vi "Set flow control 0_none.vi"(8 "error in (no error)":errorcluster caption="entrée d'erreur (pas d'erreur)", 10 "flow control (0:none)":u16(ring) items=["Aucun", "XON/XOFF", "RTS/CTS", "XON/XOFF & RTS/CTS", "DTR/DSR", "XON/XOFF & DTR/DSR"], 11 "Class Instrument UART en entrée":refnum<class "Class Instrument UART.lvclass">) -> (0 "error out":errorcluster caption="sortie d'erreur", 3 "Class Instrument UART en sortie":refnum<class "Class Instrument UART.lvclass">)   [LabVIEW 2020, in "Library Instrument & Equipement.lvlib" / "Library Instruments.lvlib" / "Class Instrument UART.lvclass"]
uses:
  Class Instrument UART.lvclass
  Class Instrument UART.lvclass/Class Instrument UART.ctl
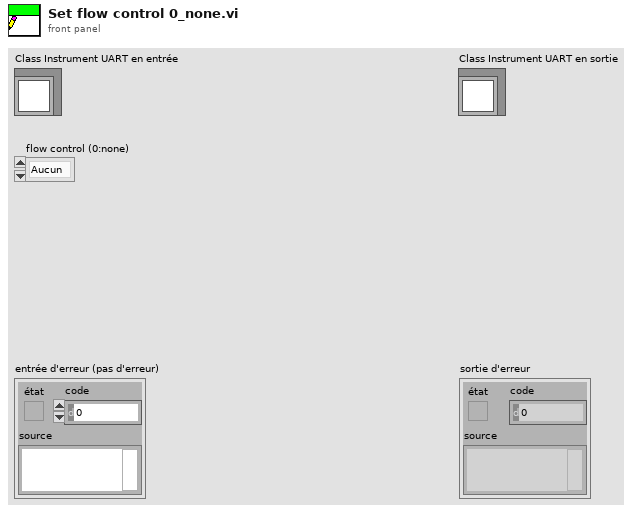
[diagram p1: front panel]
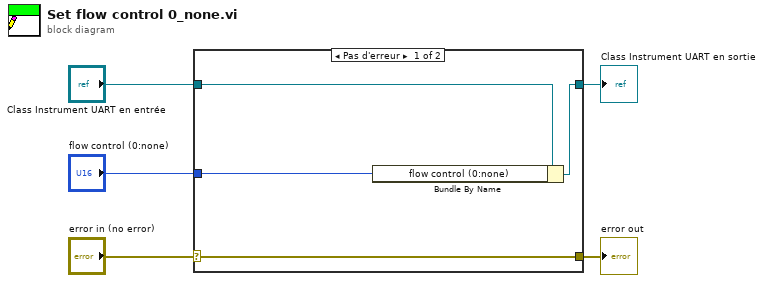
[diagram p0: block diagram]
diagram:
  n1 = case shown="Pas d'erreur" "error in (no error)" {
    selector: "error in (no error)" -> [w9 w10]
    tunnel: [w9 w10] -> w4
    tunnel: [w7 w11] -> w2
    tunnel: "Class Instrument UART en entrée" -> [w8 w11]
    tunnel: "flow control (0:none)" -> [w6 _]
    frame No Error {
      n2 = Bundle By Name(cluster=w8, "flow control (0:none)"=w6) -> (w7:refnum<class "Class Instrument UART.lvclass">)
    }
    frame Error {
    }
  }
  "error out" <- w4
  "Class Instrument UART en sortie" <- w2
